vi "Format File Header.vi"(5 "头信息数据（空）":string[](array[string]), 7 "头信息标题（空）":string[](array[string]), 8 "错误输入":cluster{"状态":bool, "代码":i32, "源":string}) -> (0 "错误输出":cluster{"状态":bool, "代码":i32, "源":string}, 3 "文件头":string)   [LabVIEW 2012]
doc: "为记录文件创建文件头。"
uses:
  <vilib>/Utility/error.llb/Error Cluster From Error Code.vi
  <vilib>/ErrorRing/Error Ring.xnode
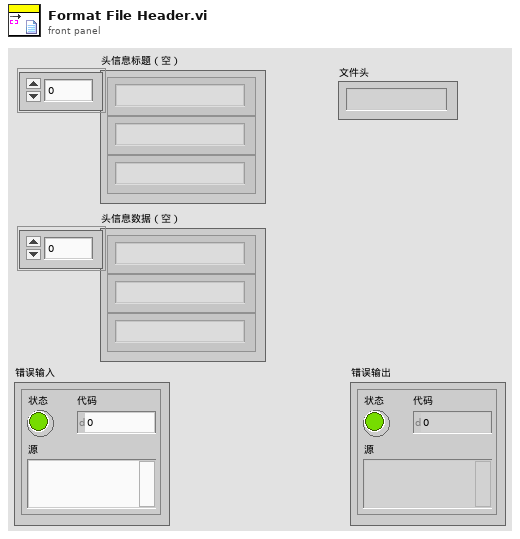
[diagram p1: front panel]
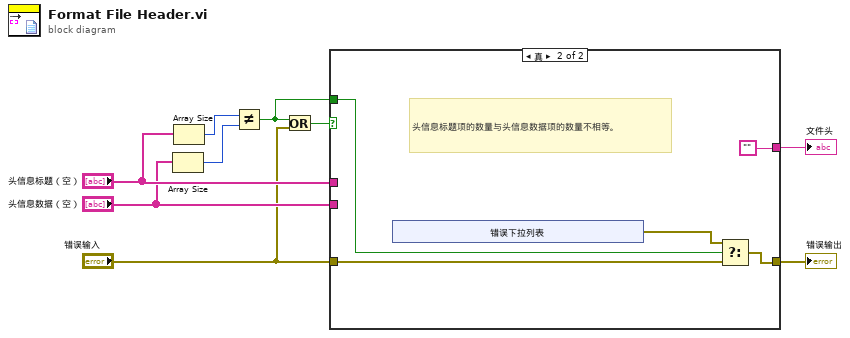
[diagram p0: block diagram]
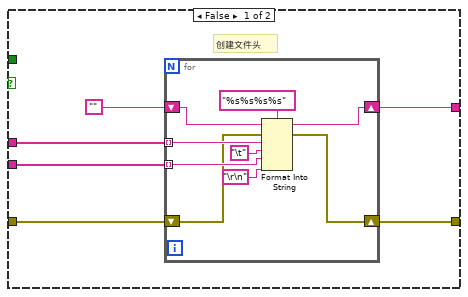
[diagram p2: hidden frame]
diagram:
  n1 = Array Size ("数组大小")(array="头信息数据（空）") -> (size(s)=w5:i32)
  n2 = Array Size ("数组大小")(array="头信息标题（空）") -> (size(s)=w6:i32)
  n3 = Not Equal? ("不等于？")(x=w6, y=w5) -> (x != y?=w2:bool)
  n4 = Or ("或")(x=w2, y="错误输入") -> (x .or. y?=w4:bool)
  n5 = case shown="真" w4 {
    tunnel: [w10 w26] -> w9
    tunnel: "头信息标题（空）" -> [w15 _]
    tunnel: "头信息数据（空）" -> [w14 _]
    tunnel: "错误输入" -> [w11 w27]
    tunnel: w2 -> [_ w28]
    tunnel: [w12 "" ("空字符串常量")] -> w1
    frame False {
      # "创建文件头"
      n6 = for {
        tunnel: w15 -> [w20] mode=indexing
        tunnel: w14 -> [w19] mode=indexing
        shift-right: [w18] -> w12
        shift-left: "" ("空字符串常量") -> [w21]
        shift-right: [w16] -> w10
        shift-left: w11 -> [w17]
        n7 = Format Into String ("格式化写入字符串")(format string="%s%s%s%s" ("格式字符串"), initial string=w21, error in=w17, w20, "\t" ("制表符常量"), w19, "\r\n" ("行结束常量")) -> (resulting string=w18:string, error out=w16:errorcluster)
      }
    }
    frame True {
      # "头信息标题项的数量与头信息数据项的数量不相等。"
      n8 = xnode "错误下拉列表"() -> ("错误输出"=w25:errorcluster)
      n9 = Select ("选择")(t=w25, s=w28, f=w27) -> (s? t:f=w26:cluster{"状态":bool, "代码":i32, "源":string})
    }
  }
  "错误输出" <- w9
  "文件头" <- w1
